vi "Read Decimation Channel.vi"(8 "error in":errorcluster, 10 "default decimation":i32=1, 11 "decimation reference in":T1 format="%.0x") -> (0 "error out":errorcluster, 3 "decimation":i32)   [LabVIEW 2019, in "Embedded Data Logger Engine.lvlib"]
uses:
  Engine/Embedded Data Logger Engine.lvlib
  <vilib>/NI VeriStand/Custom Device API/Data Reference.ctl
  <vilib>/NI VeriStand/Custom Device API/Global Data Refs.vi
  <vilib>/NI VeriStand/Custom Device API/Custom Device API.lvlib
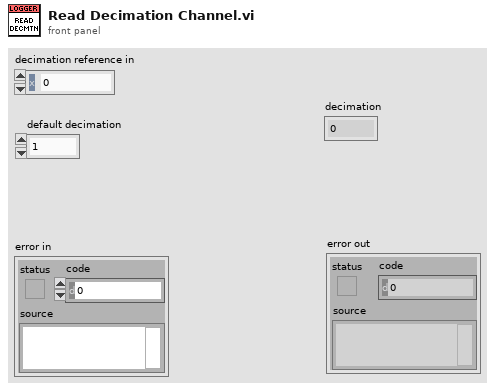
[diagram p1: front panel]
types:
  T1 = typedef "Custom Device API.lvlib/Data Reference.ctl" = i32
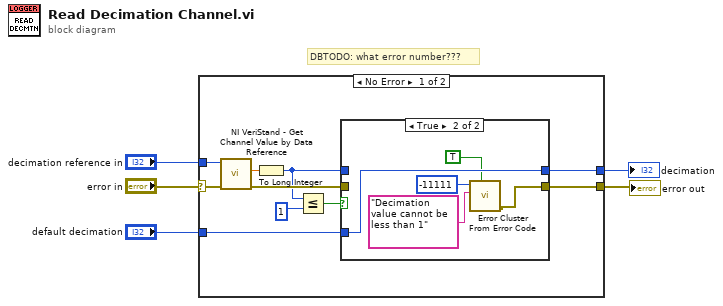
[diagram p0: block diagram]
diagram:
  # "DBTODO: what error number???"
  n1 = case shown="No Error" "error in" {
    selector: "error in" -> [w7 w24]
    tunnel: "decimation reference in" -> [w15 _]
    tunnel: "default decimation" -> [w12 w23]
    tunnel: [w10 w23] -> w3
    tunnel: [w8 w24] -> w2
    frame No Error {
      n2 = call <vilib>:"NI VeriStand - Get Channel Value by Data Reference.vi"("error in (no error)"=w7, "Data Reference in"=w15) -> ("error out"=w9:errorcluster, "Value"=w11:dbl)  [unwired: 8 in]
      n3 = To Long Integer(number=w11) -> (32bit integer=w6:i32)
      n4 = Less Or Equal?(x=w6, y=1) -> (x <= y?=w13:bool)
      n5 = case shown="True" w13 {
        tunnel: [w17 w22] -> w10
        tunnel: w12 -> [_ w22]
        tunnel: w6 -> [w17 _]
        tunnel: w9 -> [w16 _]
        tunnel: [w16 w21] -> w8
        frame False {
        }
        frame True {
          n6 = call <vilib>:"Error Cluster From Error Code.vi"("show call chain? (False)"=TRUE, "error message (\"\")"="Decimation value cannot be less than 1" ("error message (\"\")"), "error code (0)"=-11111) -> ("error out"=w21:errorcluster)  [unwired: 6 in]
        }
      }
    }
    frame Error {
    }
  }
  "decimation" <- w3
  "error out" <- w2
